vi "TrioMotion_Test3.vi"() -> ()   [LabVIEW 2020]
uses:
  aa9d9fa3-ec7e-4386-823b-d262f76d7dff.vi
  8fbe439c-06e5-460e-a560-e938ce784f44.vi
  <vilib>/Utility/inputDevices.llb/keyboardAcquire.vi
  <vilib>/Utility/inputDevices.llb/closeKeyboard.vi
panel:
  in  "Motion Tab":enum32{"POSITIONS", "PROGRAM", "AXIS ENABLE"}(tab)
  in  "Jog Axes":bool
  out "Axis Error":bool
  in  "Move":bool
  in  "Axis 2 Distance":dbl
  in  "Axis 1 Distance":dbl
  in  "Axis 0 Distance":dbl
  out "Axis 1 Endmove":dbl format="%.2g"
  out "Axis 1 Velocity":dbl format="%.2g"
  out "Axis 1 Position":dbl format="%.3g"
  out "Axis 0 Velocity":dbl format="%.2g"
  out "Axis 0 Endmove":dbl format="%.2g"
  out "Axis 0 Position":dbl format="%.3f"
  out "Axis 2 Position":dbl format="%#.3g"
  out "Axis 2 Endmove":dbl format="%#.2g"
  out "Axis 2 Velocity":dbl format="%#.2g"
  out "XY Graph":cluster{"X":dbl, "Y":dbl}[](graph)
  in  "Xmax":dbl=150.0 min=0.0 max=150.0 step=10.0
  in  "Xmin":dbl=-150.0 min=-150.0 max=0.0 step=10.0
  in  "Ymin":dbl=-150.0 min=-150.0 max=0.0 step=10.0
  in  "Ymax":dbl=150.0 min=0.0 max=150.0 step=10.0
  in  "Axis 0 Speed":dbl
  in  "Axis 1 Speed":dbl
  in  "Axis 2 Speed":dbl
  in  "Axis 1 Acc":dbl
  in  "Axis 0 Acc":dbl
  in  "Axis 2 Acc":dbl
  in  "Set Parameters 2":bool
  in  "Axis 2 Jogspeed":dbl format="%.2g"
  in  "Axis 1 Jogspeed":dbl format="%.2g"
  in  "Axis 0 Jogspeed":dbl format="%.2g"
  in  "Select Program":string(combo)="NONE"
  in  "Run Program":bool
  in  "Axis Enable":bool
  in  "?":bool
  in  "Setup Tab":enum32{"SETUP", "POWER", "ERRORS"}(tab)
  out "Loop Error":errorcluster
  out "Loop Time (us)":u32
  out "Time Elapsed (s)":i32
  out "IsOpen":bool
  in  "Connection":refnum<k7>(container)
  in  "Connect  to Controller":bool=TRUE
  in  "Set Parameters":bool
  in  "Controller Connection Type":string(combo)="2"
  out "Controller Type":string
  out "Product Name":string
  out "Version":string
  out "CommPort":fxp<+,3,3>
  # "SET PARAMETERS"
  # "DIRECT MOTION"
  # "SPEED \n(mm/s)"
  # "ACC / DEC\n(mm2/s)"
  # "JOGSPEED \n(mm/s)"
  # "Relative \n(mm)"
  # "AXIS 0"
  # "AXIS 0"
  # "AXIS 1"
  # "AXIS 1"
  # "AXIS 2"
  # "AXIS 2"
  # "FEEDBACK"
  # "AXIS\nERROR"
  # "Current Position \n(mm)"
  # "End Position \n(mm)"
  # "Velocity \n(mm2/s)"
  # "AXIS 0"
  # "AXIS 1"
  # "AXIS 2"
  # "CONTROLLER SETTINGS"
  # "ERRORS"
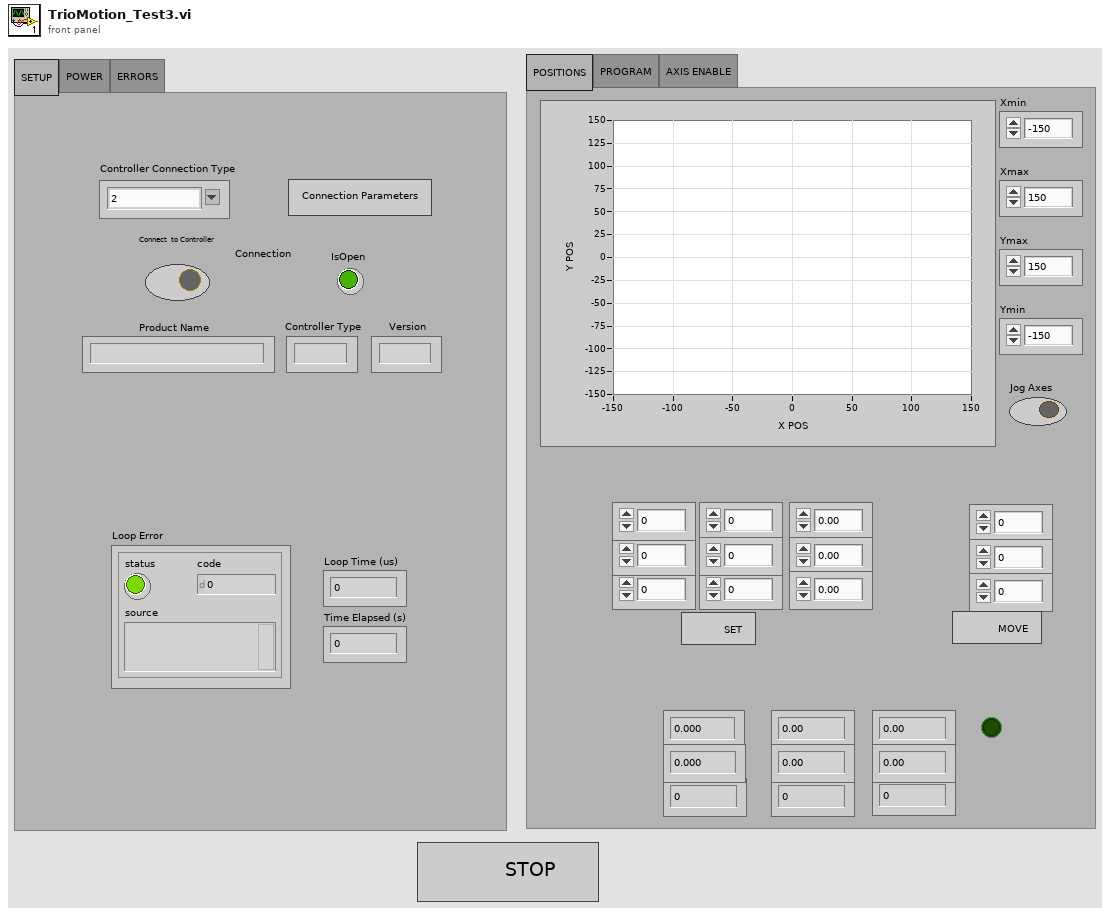
[diagram p1: front panel]
types:
  T1 = enum16{"0", "1", "2", "3", "4", "5", "6", "7", "8", "9", "A", "B", "C", "D", "E", "F", "G", "H", "I", "J", "K", "L", "M", "N", "O", "P", "Q", "R", "S", "T", "U", "V", "W", "X", "Y", "Z", "F1", "F2", "F3", "F4", "F5", "F6", "F7", "F8", "F9", "F10", "F11", "F12", "F13", "F14", "F15", "ADD", "BACK", "BACKSLASH", "CAPITAL", "COMMA", "DECIMAL", "DELETE", "DIVIDE", "DOWN", "END", "EQUALS", "ESCAPE", "GRAVE (`)", "HOME", "INSERT", "LBRACKET", "LCONTROL", "LEFT", "L ALT", "LSHIFT", "LWIN", "MINUS", "MULTIPLY", "NEXT", "NUMLOCK", "NUMPAD_0", "NUMPAD_1", "NUMPAD_2", "NUMPAD_3", "NUMPAD_4", "NUMPAD_5", "NUMPAD_6", "NUMPAD_7", "NUMPAD_8", "NUMPAD_9", "PAUSE", "PERIOD", "PRIOR (PG UP)", "RBRACKET", "RCONTROL", "RETURN", "RIGHT", "R ALT", "RSHIFT", "RWIN", "SCROLL", "SEMICOLON", "SLASH", "SPACE", "SUBTRACT", "TAB", "UP", "ENTER (num pad)", "' (quote)"}[]
  T2 = enum16{"0", "1", "2", "3", "4", "5", "6", "7", "8", "9", "A", "B", "C", "D", "E", "F", "G", "H", "I", "J", "K", "L", "M", "N", "O", "P", "Q", "R", "S", "T", "U", "V", "W", "X", "Y", "Z", "F1", "F2", "F3", "F4", "F5", "F6", "F7", "F8", "F9", "F10", "F11", "F12", "F13", "F14", "F15", "ADD", "BACK", "BACKSLASH", "CAPITAL", "COMMA", "DECIMAL", "DELETE", "DIVIDE", "DOWN", "END", "EQUALS", "ESCAPE", "GRAVE (`)", "HOME", "INSERT", "LBRACKET", "LCONTROL", "LEFT", "L ALT", "LSHIFT", "LWIN", "MINUS", "MULTIPLY", "NEXT", "NUMLOCK", "NUMPAD_0", "NUMPAD_1", "NUMPAD_2", "NUMPAD_3", "NUMPAD_4", "NUMPAD_5", "NUMPAD_6", "NUMPAD_7", "NUMPAD_8", "NUMPAD_9", "PAUSE", "PERIOD", "PRIOR (PG UP)", "RBRACKET", "RCONTROL", "RETURN", "RIGHT", "R ALT", "RSHIFT", "RWIN", "SCROLL", "SEMICOLON", "SLASH", "SPACE", "SUBTRACT", "TAB", "UP", "ENTER (num pad)", "' (quote)"}
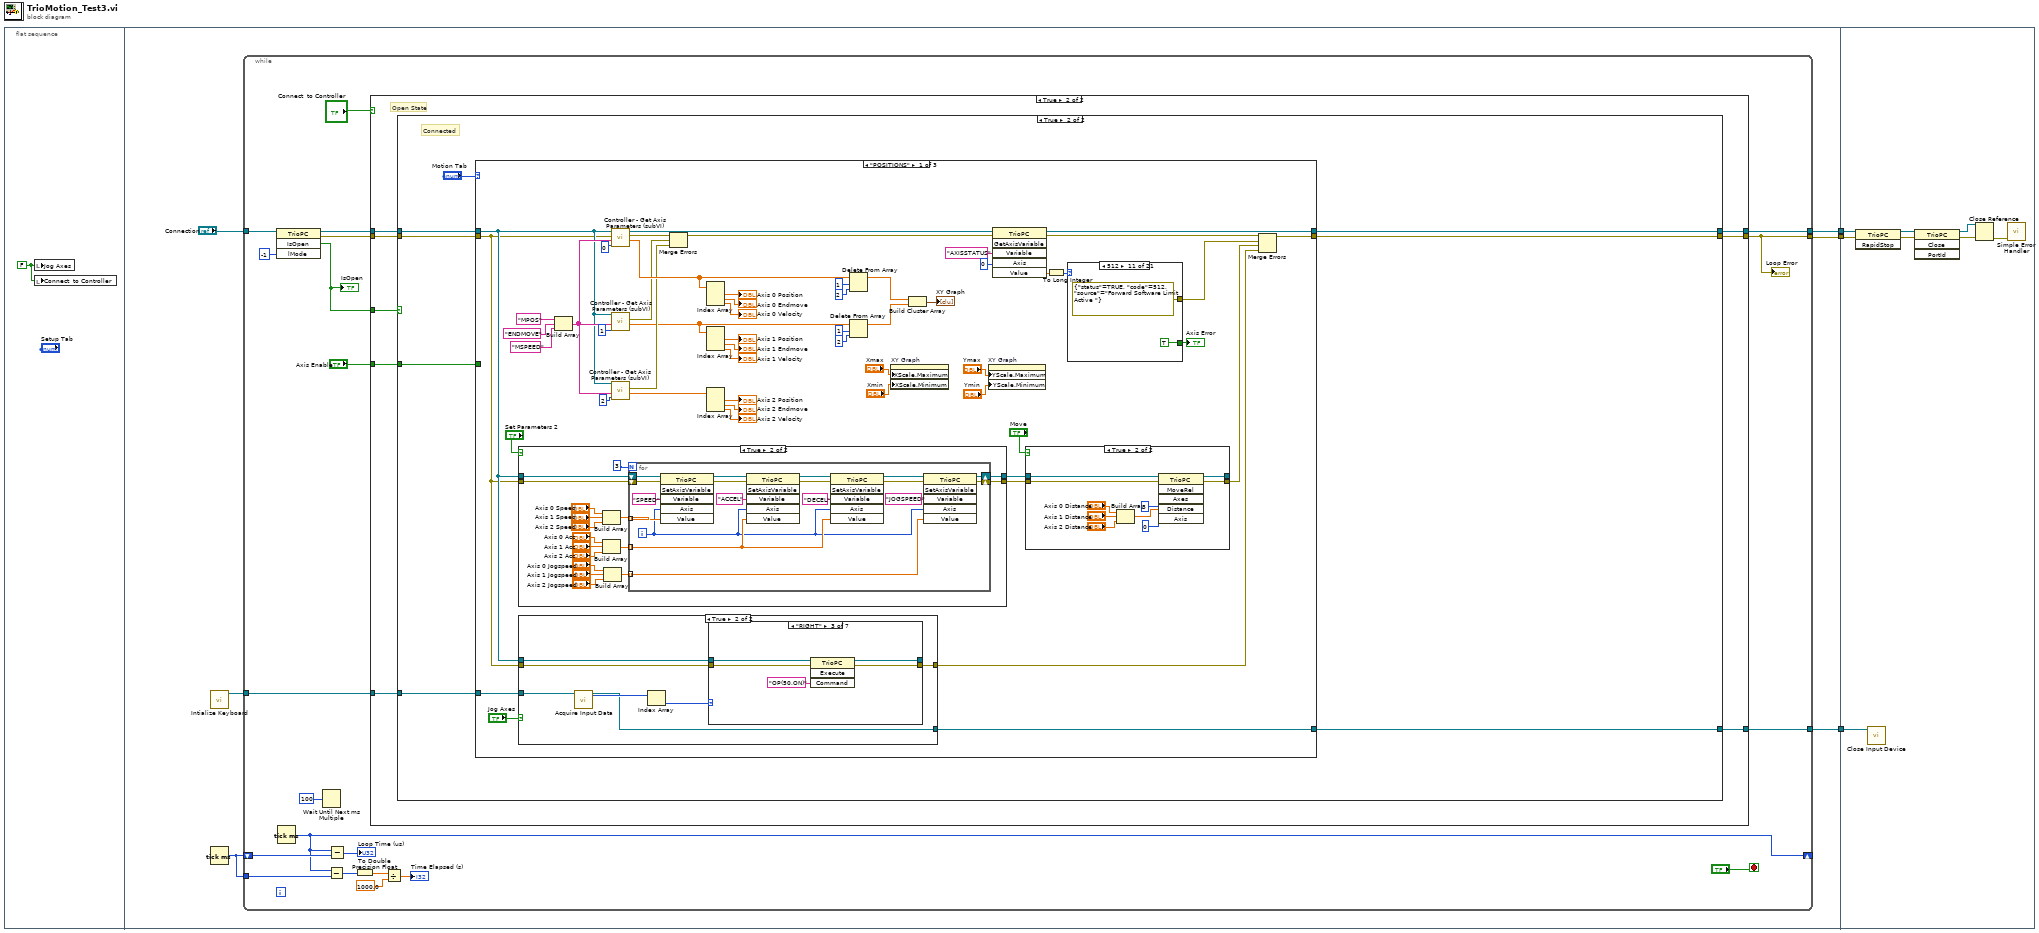
[diagram p0: block diagram]
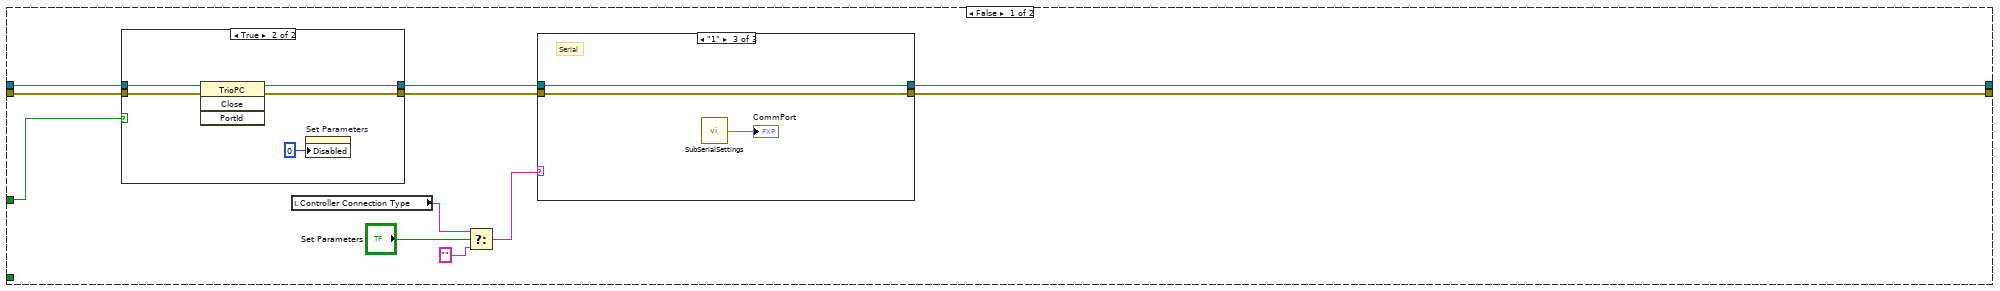
[diagram p2: hidden frame]
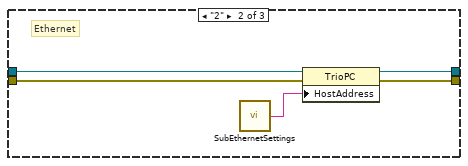
[diagram p5: hidden frame]
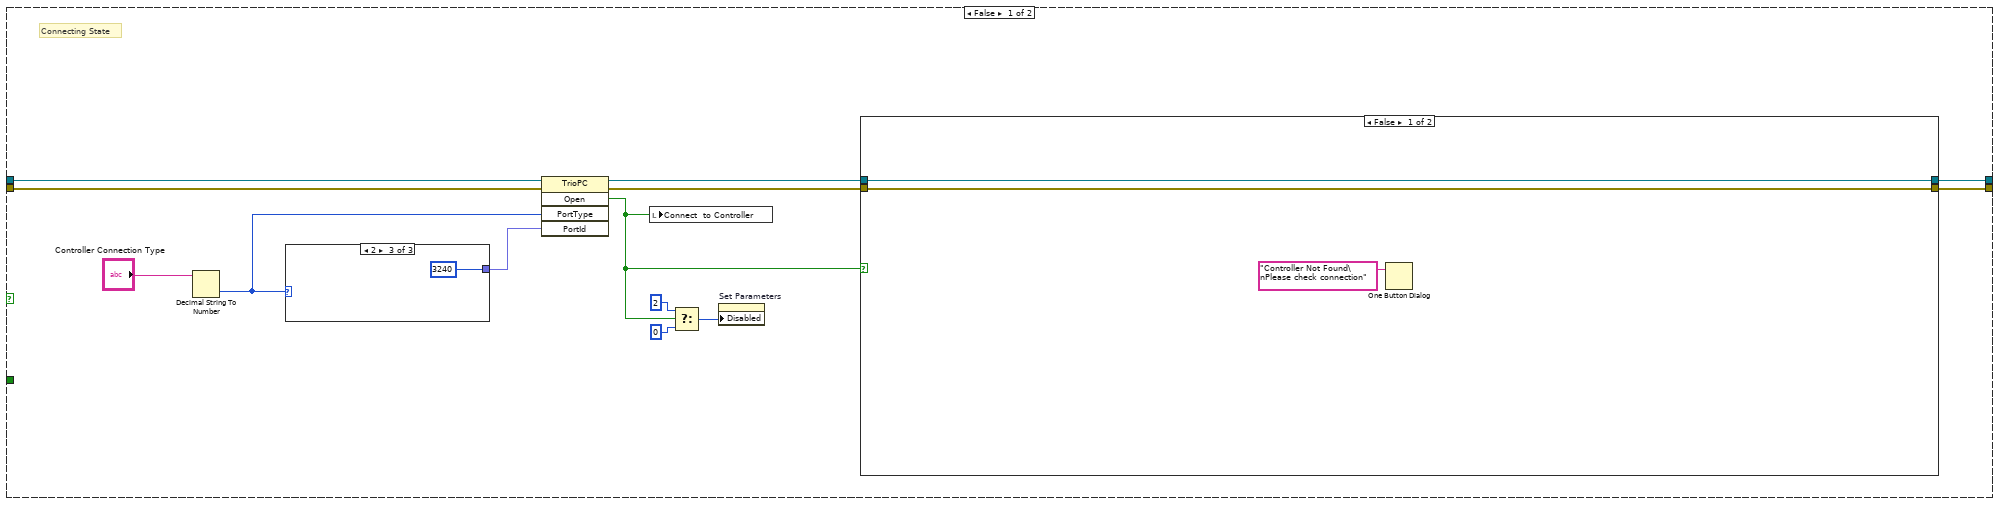
[diagram p6: hidden frame]
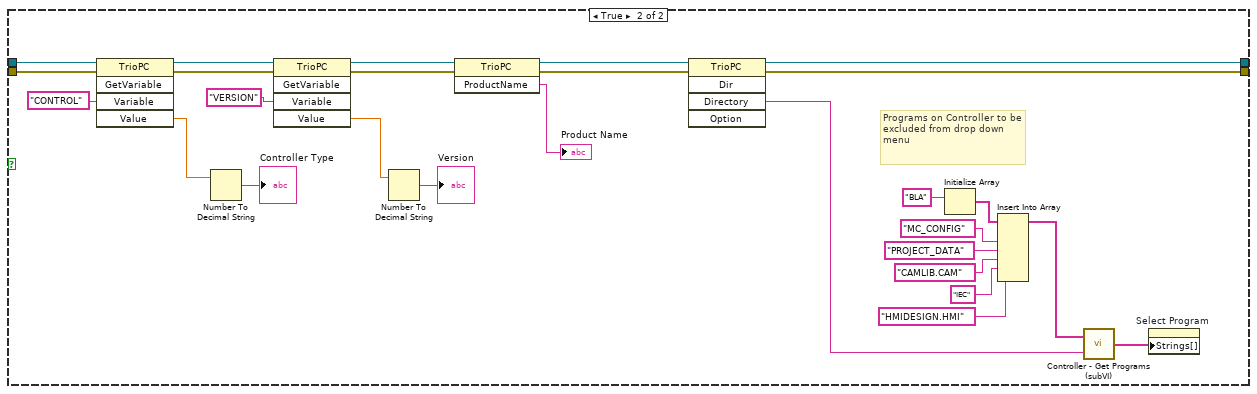
[diagram p7: hidden frame]
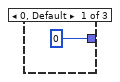
[diagram p8: hidden frame]
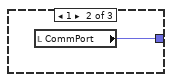
[diagram p9: hidden frame]
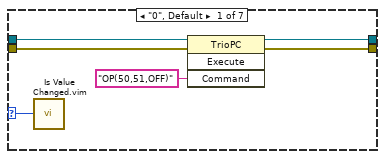
[diagram p11: hidden frame]
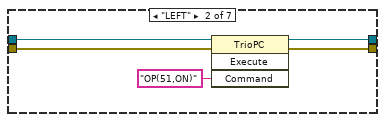
[diagram p12: hidden frame]
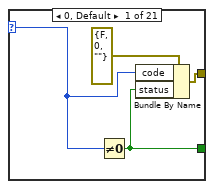
[diagram p17: hidden frame]
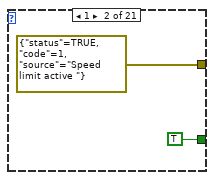
[diagram p18: hidden frame]
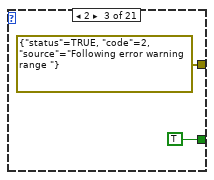
[diagram p19: hidden frame]
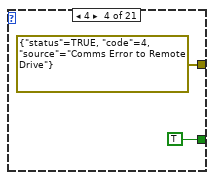
[diagram p20: hidden frame]
diagram:
  n1 = flat-sequence {
    tunnel: [w9] -> w3
    tunnel: [w8] -> w2
    tunnel: [w5] -> w1
    tunnel: w3 -> [w332]
    tunnel: w2 -> [w335]
    tunnel: w1 -> [w336]
    frame #0 {
      w4 = FALSE ("Jog Axes")
      n2 = local write "Jog Axes"(w4) -> ()
      n3 = local write "Connect  to Controller"(w4) -> ()
    }
    frame #1 {
      n4 = call <vilib>:"Intialize Keyboard.vi"() -> ("device ID"=w6:refnum<k1>)  [unwired: 1 in, 10 out]
      n5 = Tick Count (ms)() -> (millisecond timer value=w7:u32)
      n6 = while {
        tunnel: "Connection" -> [w29]
        tunnel: [w26] -> w9
        tunnel: [w15] -> w8
        shift-right: [w18] -> _
        shift-left: w7 -> [w22]
        tunnel: w7 -> [w17]
        tunnel: w6 -> [w14]
        tunnel: [w13] -> w5
        stop <- "?" stop-if-true
        n7 = invoke class="TrioPC" method="IsOpen"(reference=w29, "lMode"=-1) -> (reference out=w12:refnum<k7>, error out=w11:errorcluster, "IsOpen"=w27:bool)  [unwired: 2 in, 1 out]
        "IsOpen" <- w27
        n8 = Tick Count (ms)() -> (millisecond timer value=w18:u32)
        n9 = Wait Until Next ms Multiple(millisecond multiple=u32 100) -> ()  [unwired: 1 out]
        n10 = Subtract(x=w18, y=w17) -> (x-y=w16:u32)
        n11 = Subtract(x=w18, y=w22) -> (x-y=→"Loop Time (us)":u32)
        n12 = To Double Precision Float(number=w16) -> (double precision float=w19:dbl)
        n13 = case shown="True" "Connect  to Controller" {
          tunnel: [w36 w67] -> w26
          tunnel: [w37 w66] -> w15
          tunnel: w27 -> [w33 w65]
          tunnel: w12 -> [w35 w64]
          tunnel: w11 -> [w34 w63]
          tunnel: "Axis Enable" -> [_ w62]
          tunnel: w14 -> [_ w61]
          tunnel: [_ w60] -> w13
          frame False {
            n14 = case shown="True" w33 {
              tunnel: [w44 w49] -> w39
              tunnel: [w43 w48] -> w38
              tunnel: w35 -> [w44 w46]
              tunnel: w34 -> [w43 w45]
              frame False {
              }
              frame True {
                n15 = invoke class="TrioPC" method="Close"(reference=w46, error in=w45) -> (reference out=w49:refnum<k7>, error out=w48:errorcluster)  [unwired: 2 in, 2 out]
                n16 = property on="Set Parameters" class="Bool"("Disabled"=u8 0) -> ()  [unwired: 2 in, 2 out]
              }
            }
            n17 = local read "Controller Connection Type"() -> (w32:string)
            n18 = Select(t=w32, s="Set Parameters", f="") -> (s? t:f=w40:string)
            n19 = case shown="\"1\"" w40 {
              tunnel: w39 -> [w51 w54 w59]
              tunnel: w38 -> [w50 w53 w58]
              tunnel: [w51 w56 w59] -> w36
              tunnel: [w50 w55 w58] -> w37
              frame "", Default {
              }
              frame "2" {
                # "Ethernet"
                n20 = call "SubEthernetSettings.vi"() -> ("Ethernet IP Address 2"=w52:string)
                n21 = property class="TrioPC"(reference=w54, error in=w53, "HostAddress"=w52) -> (reference out=w56:refnum<k7>, error out=w55:errorcluster)
              }
              frame "1" {
                # "Serial"
                n22 = call "SubSerialSettings.vi"() -> ("CommPort"=→"CommPort":fxp<+,3,3>)
              }
            }
          }
          frame True {
            # "Open State"
            n23 = case shown="True" w65 {
              tunnel: [w71 w117] -> w67
              tunnel: [w72 w116] -> w66
              tunnel: w64 -> [w76 w118]
              tunnel: w63 -> [w75 w119]
              tunnel: w62 -> [_ w121]
              tunnel: w61 -> [_ w115]
              tunnel: [_ w114] -> w60
              frame False {
                # "Connecting State"
                n24 = Decimal String To Number(string="Controller Connection Type") -> (number=w73:i32)  [unwired: 2 in, 1 out]
                n25 = case shown="2" w73 {
                  tunnel: [i16 0 ("PortId") w112 i16 3240 ("PortId")] -> w80
                  frame 0, Default {
                  }
                  frame 1 {
                    n26 = local read "CommPort"() -> (w112:fxp<+,3,3>)
                  }
                  frame 2 {
                  }
                }
                n27 = invoke class="TrioPC" method="Open"(reference=w76, error in=w75, "PortType"=w73, "PortId"=w80) -> (reference out=w70:refnum<k7>, error out=w69:errorcluster, "Open"=w68:bool)  [unwired: 1 in, 2 out]
                n28 = local write "Connect  to Controller"(w68) -> ()
                n29 = Select(t=u8 2, s=w68, f=u8 0 ("Disabled")) -> (s? t:f=w77:u8)
                n30 = property on="Set Parameters" class="Bool"("Disabled"=w77) -> ()  [unwired: 2 in, 2 out]
                n31 = case shown="False" w68 {
                  tunnel: [w82 w108] -> w72
                  tunnel: [w83 w107] -> w71
                  tunnel: w70 -> [w83 w98]
                  tunnel: w69 -> [w82 w89]
                  frame False {
                    n32 = One Button Dialog(message="Controller Not Found\nPlease check connection") -> ()  [unwired: 1 in, 1 out]
                  }
                  frame True {
                    # "Programs on Controller to be excluded from drop down menu"
                    n33 = invoke class="TrioPC" method="GetVariable"(reference=w98, error in=w89, "Variable"="CONTROL") -> (reference out=w91:refnum<k7>, error out=w90:errorcluster, "Value"=w95:dbl)  [unwired: 2 in, 2 out]
                    n34 = Number To Decimal String(number=w95) -> (decimal integer string=→"Controller Type":string)  [unwired: 1 in]
                    n35 = invoke class="TrioPC" method="GetVariable"(reference=w91, error in=w90, "Variable"="VERSION") -> (reference out=w87:refnum<k7>, error out=w88:errorcluster, "Value"=w94:dbl)  [unwired: 2 in, 2 out]
                    n36 = Number To Decimal String(number=w94) -> (decimal integer string=→"Version":string)  [unwired: 1 in]
                    n37 = invoke class="TrioPC" method="ProductName"(reference=w87, error in=w88) -> (reference out=w86:refnum<k7>, error out=w85:errorcluster, "ProductName"=→"Product Name":string)  [unwired: 1 in]
                    n38 = invoke class="TrioPC" method="Dir"(reference=w86, error in=w85) -> (reference out=w107:refnum<k7>, error out=w108:errorcluster, "Directory"=w109:string)  [unwired: 3 in, 2 out]
                    n39 = Initialize Array("BLA" ("element")) -> (w106:string[])  [unwired: 1 in]
                    n40 = Insert Into Array(array=w106, new element #1="MC_CONFIG" ("element"), new element #2="PROJECT_DATA" ("element"), new element #3="CAMLIB.CAM" ("element"), new element #4="IEC" ("element"), new element #5="HMIDESIGN.HMI") -> (w99:string[])  [unwired: 1 in]
                    n41 = call "Controller - Get Programs (subVI).vi"("Controller Directory"=w109, "Exclusion List"=w99) -> ("Programs List"=w110:string[])
                    n42 = property on="Select Program" class="CmbBox"("Strings[]"=w110) -> ()  [unwired: 2 in, 2 out]
                  }
                }
              }
              frame True {
                # "Connected"
                n43 = case shown="\"POSITIONS\"" "Motion Tab" {
                  tunnel: w119 -> [w136 w300 w312]
                  tunnel: [w135 w299 w310] -> w116
                  tunnel: w118 -> [w137 w298 w311]
                  tunnel: [w131 w297 w309] -> w117
                  tunnel: w121 -> [_ _ w308]
                  tunnel: w115 -> [w139 _ _]
                  tunnel: [w138 _ _] -> w114
                  frame "POSITIONS" {
                    n44 = case shown="True" "Set Parameters 2" {
                      tunnel: [w246 w255] -> w141
                      tunnel: w137 -> [w247 w250]
                      tunnel: w136 -> [w246 w249]
                      tunnel: [w247 w248] -> w142
                      frame False {
                      }
                      frame True {
                        n45 = Build Array("Axis 0 Speed", "Axis 1 Speed", "Axis 2 Speed") -> (w261:dbl[])
                        n46 = Build Array("Axis 0 Acc", "Axis 1 Acc", "Axis 2 Acc") -> (w260:dbl[])
                        n47 = Build Array("Axis 0 Jogspeed", "Axis 1 Jogspeed", "Axis 2 Jogspeed") -> (w251:dbl[])
                        n48 = for {
                          N: 3 -> [_]
                          tunnel: w261 -> [w273] mode=indexing
                          tunnel: w260 -> [w272] mode=indexing
                          tunnel: w251 -> [w274] mode=indexing
                          shift-right: [w265] -> w255
                          shift-left: w249 -> [w269]
                          shift-right: [w266] -> w248
                          shift-left: w250 -> [w270]
                          i -> [w271]
                          n49 = invoke class="TrioPC" method="SetAxisVariable"(reference=w270, error in=w269, "Variable"="SPEED", "Axis"=w271, "Value"=w273) -> (reference out=w281:refnum<k7>, error out=w280:errorcluster)  [unwired: 1 in, 4 out]
                          n50 = invoke class="TrioPC" method="SetAxisVariable"(reference=w281, error in=w280, "Variable"="ACCEL", "Axis"=w271, "Value"=w272) -> (reference out=w279:refnum<k7>, error out=w278:errorcluster)  [unwired: 1 in, 4 out]
                          n51 = invoke class="TrioPC" method="SetAxisVariable"(reference=w279, error in=w278, "Variable"="DECEL", "Axis"=w271, "Value"=w272) -> (reference out=w268:refnum<k7>, error out=w267:errorcluster)  [unwired: 1 in, 4 out]
                          n52 = invoke class="TrioPC" method="SetAxisVariable"(reference=w268, error in=w267, "Variable"="JOGSPEED", "Axis"=w271, "Value"=w274) -> (reference out=w266:refnum<k7>, error out=w265:errorcluster)  [unwired: 1 in, 4 out]
                        }
                      }
                    }
                    n53 = case shown="True" "Jog Axes" {
                      tunnel: w139 -> [w177 w183]
                      tunnel: [w177 w182] -> w138
                      tunnel: w137 -> [_ w181]
                      tunnel: w136 -> [w178 w180]
                      tunnel: [w178 w179] -> w124
                      frame False {
                      }
                      frame True {
                        n54 = call-poly <vilib>:"Acquire Input Data.vi"("device ID"=w183) -> ("device ID"=w182:refnum<k1>, "keys pressed"=w185:T1)  [unwired: 1 in, 16 out]
                        n55 = Index Array(array=w185) -> (element=w184:T2)  [unwired: 1 in]
                        n56 = case shown="\"RIGHT\"" w184 {
                          selector: w184 -> [w187 _ _ _ _ _ _]
                          tunnel: w181 -> [w191 w195 w201 _ _ _ _]
                          tunnel: w180 -> [w190 w196 w200 _ _ _ _]
                          tunnel: [w189 w194 w199 _ _ _ _] -> _
                          tunnel: [w188 w193 w198 _ _ _ _] -> w179
                          frame "0", Default {
                            n57 = call "Is Value Changed.vim"("value"=w187) -> ()  [unwired: 1 out]
                            n58 = invoke class="TrioPC" method="Execute"(reference=w191, error in=w190, "Command"="OP(50,51,OFF)") -> (reference out=w189:refnum<k7>, error out=w188:errorcluster)  [unwired: 1 in, 2 out]
                          }
                          frame "LEFT" {
                            n59 = invoke class="TrioPC" method="Execute"(reference=w195, error in=w196, "Command"="OP(51,ON)") -> (reference out=w194:refnum<k7>, error out=w193:errorcluster)  [unwired: 1 in, 2 out]
                          }
                          frame "RIGHT" {
                            n60 = invoke class="TrioPC" method="Execute"(reference=w201, error in=w200, "Command"="OP(50,ON)") -> (reference out=w199:refnum<k7>, error out=w198:errorcluster)  [unwired: 1 in, 2 out]
                          }
                          frame "UP" {
                          }
                          frame "DOWN" {
                          }
                          frame "PRIOR (PG UP)" {
                          }
                          frame "NEXT" {
                          }
                        }
                      }
                    }
                    n61 = Build Array("MPOS", "ENDMOVE", "MSPEED") -> (w154:string[])
                    n62 = call "Controller - Get Axis Parameters (subVI).vi"("Axis"=i16 2, "Axis Parameters"=w154, "Automation Refnum in"=w137) -> ("Axis Parameter Values"=w153:dbl[], "error out"=w145:errorcluster)  [unwired: 6 in, 1 out]
                    n63 = call "Controller - Get Axis Parameters (subVI).vi"("Axis"=i16 0, "Axis Parameters"=w154, "error in (no error)"=w136, "Automation Refnum in"=w137) -> ("Axis Parameter Values"=w150:dbl[], "error out"=w147:errorcluster, "Automation Refnum out"=w130:refnum<k7>)  [unwired: 5 in]
                    n64 = call "Controller - Get Axis Parameters (subVI).vi"("Axis"=i16 1, "Axis Parameters"=w154, "Automation Refnum in"=w137) -> ("Axis Parameter Values"=w144:dbl[], "error out"=w146:errorcluster)  [unwired: 6 in, 1 out]
                    n65 = Merge Errors(w147, w146, w145) -> (w129:errorcluster)
                    n66 = Index Array(array=w150) -> (element #1=→"Axis 0 Position":dbl, element #2=→"Axis 0 Endmove":dbl, element #3=→"Axis 0 Velocity":dbl)  [unwired: 3 in]
                    n67 = Index Array(array=w144) -> (element #1=→"Axis 1 Position":dbl, element #2=→"Axis 1 Endmove":dbl, element #3=→"Axis 1 Velocity":dbl)  [unwired: 3 in]
                    n68 = Index Array(array=w153) -> (element #1=→"Axis 2 Position":dbl, element #2=→"Axis 2 Endmove":dbl, element #3=→"Axis 2 Velocity":dbl)  [unwired: 3 in]
                    n69 = Delete From Array(array=w150, length=1, index=2) -> (array with subset deleted=w170:dbl[])  [unwired: 1 out]
                    n70 = Delete From Array(array=w144, length=1, index=2) -> (array with subset deleted=w163:dbl[])  [unwired: 1 out]
                    n71 = property on="XY Graph" class="XYGraph (strict)"("XScale.Maximum"="Xmax", "XScale.Minimum"="Xmin") -> ()  [unwired: 2 in, 2 out]
                    n72 = Build Cluster Array(w170, w163) -> (→"XY Graph":cluster{dbl, dbl}[])
                    n73 = property on="XY Graph" class="XYGraph (strict)"("YScale.Maximum"="Ymax", "YScale.Minimum"="Ymin") -> ()  [unwired: 2 in, 2 out]
                    n74 = invoke class="TrioPC" method="GetAxisVariable"(reference=w130, error in=w129, "Variable"="AXISSTATUS", "Axis"=i16 0) -> (reference out=w131:refnum<k7>, error out=w132:errorcluster, "Value"=w128:dbl)  [unwired: 2 in, 3 out]
                    n75 = case shown="True" "Move" {
                      tunnel: [w284 w288] -> _
                      tunnel: [w283 w287] -> w123
                      tunnel: w142 -> [w284 w286]
                      tunnel: w141 -> [w283 w285]
                      frame False {
                      }
                      frame True {
                        n76 = Build Array("Axis 0 Distance", "Axis 1 Distance", "Axis 2 Distance") -> (w292:dbl[])
                        n77 = invoke class="TrioPC" method="MoveRel"(reference=w286, error in=w285, "Axes"=i16 3, "Distance"=w292, "Axis"=0) -> (reference out=w288:refnum<k7>, error out=w287:errorcluster)  [unwired: 1 in, 4 out]
                      }
                    }
                    n78 = To Long Integer(number=w128) -> (32bit integer=w127:i32)
                    n79 = case shown="512" w127 {
                      selector: w127 -> [w202 _ _ _ _ _ _ _ _ _ _ _ _ _ _ _ _ _ _ _ _]
                      tunnel: [w203 TRUE TRUE TRUE TRUE TRUE TRUE FALSE TRUE TRUE TRUE TRUE FALSE TRUE TRUE TRUE TRUE TRUE TRUE TRUE TRUE] -> w126
                      tunnel: [w204 errorcluster {"status"=TRUE, "code"=1, "source"="Speed limit active "} ("error in (no error)") errorcluster {"status"=TRUE, "code"=2, "source"="Following error warning range "} ("error in (no error)") errorcluster {"status"=TRUE, "code"=4, "source"="Comms Error to Remote Drive"} ("error in (no error)") errorcluster {"status"=TRUE, "code"=8, "source"="Remote drive error"} ("error in (no error)") errorcluster {"status"=TRUE, "code"=16, "source"="Forward hardware limit "} ("error in (no error)") errorcluster {"status"=TRUE, "code"=32, "source"="Reverse hardware limit "} ("error in (no error)") errorcluster {"status"=FALSE, "code"=64, "source"="Datuming in Progress"} ("error in (no error)") errorcluster {"status"=TRUE, "code"=128, "source"="Feedhold Active"} ("error in (no error)") errorcluster {"status"=TRUE, "code"=256, "source"="Following Error Exceeds Limit"} ("error in (no error)") errorcluster {"status"=TRUE, "code"=512, "source"="Forward Software Limit Active "} ("error in (no error)") errorcluster {"status"=TRUE, "code"=1024, "source"="Reverse Software Limit Active "} ("error in (no error)") errorcluster {"status"=FALSE, "code"=2048, "source"="Cancelling the move "} ("error in (no error)") errorcluster {"status"=TRUE, "code"=4096, "source"="Pulse Output Axis Oxer-Speed"} ("error in (no error)") errorcluster {"status"=TRUE, "code"=8192, "source"="MOVETANG Decelerating"} ("error in (no error)") errorcluster {"status"=TRUE, "code"=32768, "source"="VOLUME_LIMIT Active"} ("error in (no error)") errorcluster {"status"=TRUE, "code"=65536, "source"="AXIS_FS_LIMIT Active"} ("error in (no error)") errorcluster {"status"=TRUE, "code"=131072, "source"="AXIS_RS_LIMIT Active"} ("error in (no error)") errorcluster {"status"=TRUE, "code"=262144, "source"="Encoder Power Supply Overload"} ("error in (no error)") errorcluster {"status"=TRUE, "code"=524288, "source"="HW_PSWITCH FIFO Not Empty"} ("error in (no error)") errorcluster {"status"=TRUE, "code"=1048576, "source"="HW_PSWITCH FIFO Full"} ("error in (no error)")] -> w125
                      frame 0, Default {
                        n80 = Not Equal To 0?(x=w202) -> (x != 0?=w203:bool)
                        n81 = Bundle By Name(cluster=errorcluster {"status"=FALSE, "code"=0, "source"=""} ("error in (no error)"), "code"=w202, "status"=w203) -> (w204:errorcluster)
                      }
                      frame 1 {
                      }
                      frame 2 {
                      }
                      frame 4 {
                      }
                      frame 8 {
                      }
                      frame 16 {
                      }
                      frame 32 {
                      }
                      frame 64 {
                      }
                      frame 128 {
                      }
                      frame 256 {
                      }
                      frame 512 {
                      }
                      frame 1024 {
                      }
                      frame 2048 {
                      }
                      frame 4096 {
                      }
                      frame 8192 {
                      }
                      frame 32768 {
                      }
                      frame 65536 {
                      }
                      frame 131072 {
                      }
                      frame 262144 {
                      }
                      frame 524288 {
                      }
                      frame 1048576 {
                      }
                    }
                    "Axis Error" <- w126
                    n82 = Merge Errors(w132, w125, w123, w124) -> (w135:errorcluster)
                  }
                  frame "PROGRAM" {
                    n83 = case shown="True" "Run Program" {
                      tunnel: "Select Program" -> [_ w307]
                      tunnel: w300 -> [w302 w306]
                      tunnel: [w302 w305] -> w299
                      tunnel: w298 -> [w301 w304]
                      tunnel: [w301 w303] -> w297
                      frame False {
                      }
                      frame True {
                        n84 = invoke class="TrioPC" method="Run"(reference=w304, error in=w306, "Program"=w307) -> (reference out=w303:refnum<k7>, error out=w305:errorcluster)  [unwired: 2 in, 3 out]
                      }
                    }
                  }
                  frame "AXIS ENABLE", Default {
                    n85 = call "Is Value Changed.vim"("value"=w308) -> ("changed or first call?"=w313:bool)
                    n86 = case shown="True" w313 {
                      tunnel: [w315 w320] -> w310
                      tunnel: w312 -> [w315 w319]
                      tunnel: w311 -> [w314 w318]
                      tunnel: [w314 w317] -> w309
                      tunnel: w308 -> [_ w316]
                      frame False {
                      }
                      frame True {
                        n87 = case shown="False" w316 {
                          tunnel: [w325 w330] -> w320
                          tunnel: w319 -> [w324 w329]
                          tunnel: w318 -> [w323 w328]
                          tunnel: [w322 w327] -> w317
                          frame False {
                            n88 = invoke class="TrioPC" method="Run"(reference=w323, error in=w324, "Program"="AXIS_DISABLE") -> (reference out=w322:refnum<k7>, error out=w325:errorcluster)  [unwired: 2 in, 3 out]
                          }
                          frame True {
                            n89 = invoke class="TrioPC" method="Run"(reference=w328, error in=w329, "Program"="AXIS_ENABLE") -> (reference out=w327:refnum<k7>, error out=w330:errorcluster)  [unwired: 2 in, 3 out]
                          }
                        }
                      }
                    }
                  }
                }
              }
            }
          }
        }
        "Loop Error" <- w15
        n90 = Divide(x=w19, y=1000.0) -> (x/y=→"Time Elapsed (s)":dbl)
      }
    }
    frame #2 {
      n91 = invoke class="TrioPC" method="RapidStop"(reference=w332, error in=w335) -> (reference out=w333:refnum<k7>, error out=w334:errorcluster)  [unwired: 1 in, 1 out]
      n92 = call-poly <vilib>:"Close Input Device.vi"("device ID"=w336) -> ()  [unwired: 9 in, 1 out]
      n93 = invoke class="TrioPC" method="Close"(reference=w333, error in=w334) -> (reference out=w337:refnum<k7>, error out=w338:errorcluster)  [unwired: 2 in, 2 out]
      n94 = Close Reference(reference=w337, error in (no error)=w338) -> (error out=w331:errorcluster)
      n95 = call <vilib>:"Simple Error Handler.vi"("error in (no error)"=w331) -> ()  [unwired: 4 in, 5 out]
    }
  }
